vi "Clear.vi"(8 "error in (no error)":errorcluster, 11 "Execution API In":refnum<class "Execution API.lvclass">) -> (0 "error out":errorcluster, 3 "Execution API Out":refnum<class "Execution API.lvclass">)   [LabVIEW 2020, in "Execution API.lvclass"]
doc: "Clears any resorces allocated during initialization."
uses:
  Execution API.lvclass
  Process/Process.lvclass
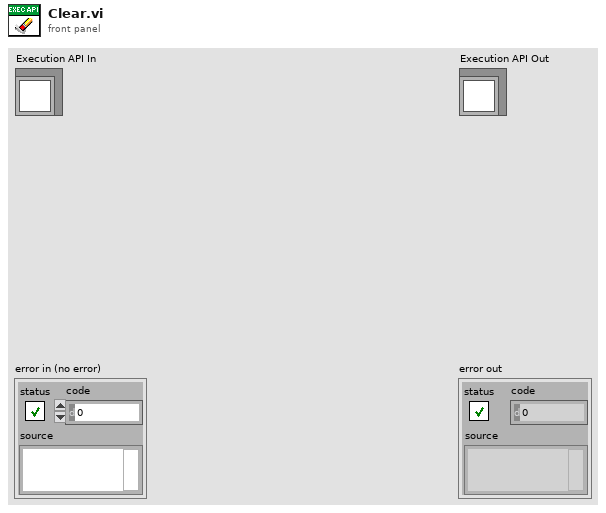
[diagram p1: front panel]
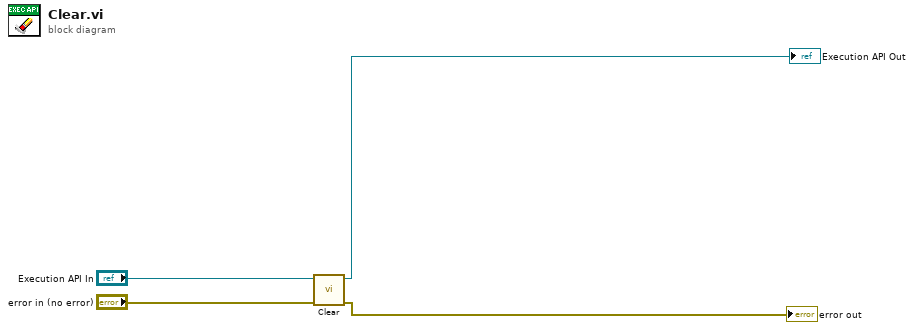
[diagram p0: block diagram]
diagram:
  n1 = call-parent "Clear.vi"("error in (no error)"="error in (no error)", "Process In"="Execution API In") -> ("error out"=→"error out":errorcluster, "Process Out"=→"Execution API Out":refnum<class "Execution API.lvclass">)  [unwired: 8 in]
